vi "Set configuration chain.vi"(8 "error in (no error)":errorcluster, 9 "class names":string[](array[string]), 10 "configuration":variant[](array[variant]), 11 "ExampleClassA in":refnum<class "ExampleClassA.lvclass">) -> (0 "error out":errorcluster, 3 "ExampleClassA out":refnum<class "ExampleClassA.lvclass">)   [LabVIEW 2012, in "ExampleClassA.lvclass"]
uses:
  ExampleClassA.lvclass
  <vilib>/Distrio/Murmex/Murmex/Murmex.lvclass
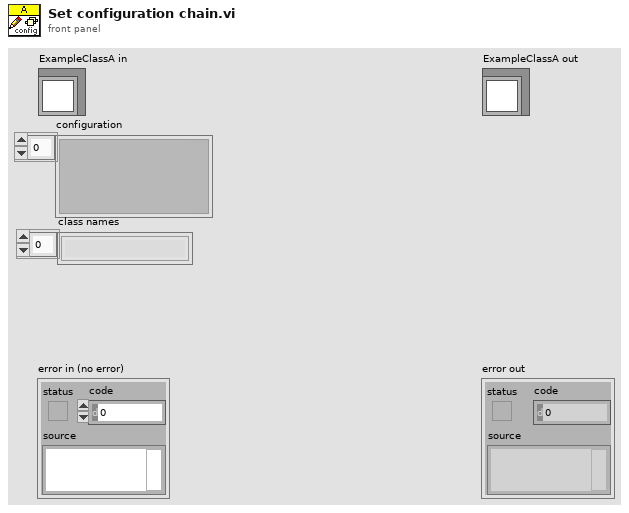
[diagram p1: front panel]
types:
  T1 = typedef "ExampleClassA.lvclass/Settings cluster.ctl" = cluster{"period?":dbl[unit], "number of blocks":i32, "number of channels":i32}
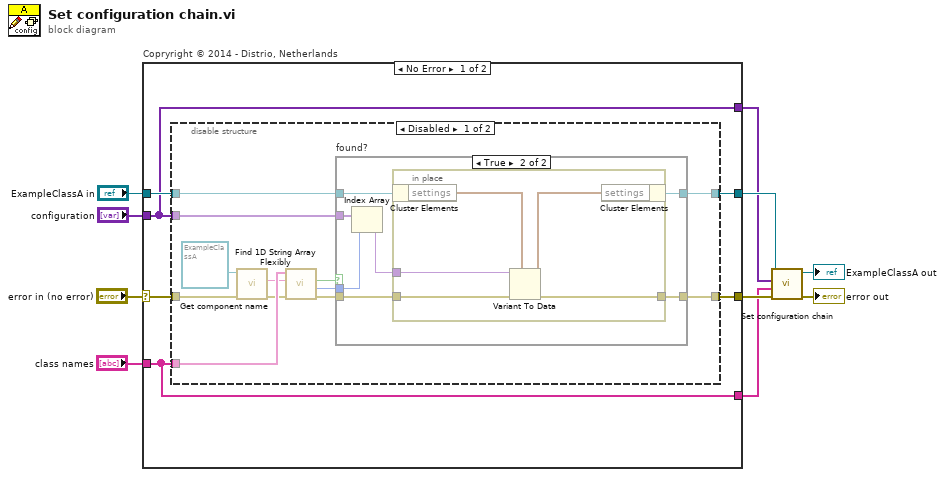
[diagram p0: block diagram]
diagram:
  n1 = case "Copryright © 2014 - Distrio, Netherlands" shown="No Error" "error in (no error)" {
    selector: "error in (no error)" -> [w16 w48]
    tunnel: [w13 w48] -> w8
    tunnel: [w14 w47] -> w3
    tunnel: "ExampleClassA in" -> [w15 w47]
    tunnel: "class names" -> [w11 w45]
    tunnel: "configuration" -> [w12 w46]
    tunnel: [w12 w46] -> w2
    tunnel: [w11 w45] -> w1
    frame No Error {
      n2 = disable-structure shown="Disabled" {
        disable-tunnel: w16 -> [w28 w43]
        disable-tunnel: w15 -> [w18 w44]
        disable-tunnel: [w27 w44] -> w14
        disable-tunnel: [w26 w43] -> w13
        disable-tunnel: w12 -> [w25 _]
        disable-tunnel: w11 -> [w24 _]
        frame Disabled {
          n3 = call <vilib>:"Get component name.vi"("error in (no error)"=w28, "Murmex in"=refnum<class "ExampleClassA.lvclass"> refnum ("ExampleClassA")) -> ("error out"=w22:errorcluster, "component name"=w23:string)  [unwired: 7 in, 1 out]
          n4 = call <vilib>:"Find 1D String Array Flexibly.vi"("error in (no error)"=w22, "element"=w23, "array"=w24) -> ("error out"=w21:errorcluster, "index of element"=w20:i32, "found?"=w19:bool)  [unwired: 6 in]
          n5 = case "found?" shown="True" w19 {
            tunnel: w18 -> [w29 w36]
            tunnel: [w29 w35] -> w27
            tunnel: [w30 w34] -> w26
            tunnel: w25 -> [_ w33]
            tunnel: w21 -> [w30 w32]
            tunnel: w20 -> [_ w31]
            frame False {
            }
            frame True {
              n6 = Index Array(array=w33, index=w31) -> (element=w37:variant)
              n7 = in-place {
                in-place-border: w37 -> [w42]
                in-place-border: w32 -> [w40]
                in-place-border: [w38] -> w34
                n8 = in-place-cluster #1(w36) -> ("settings"=w41:T1)
                n9 = Variant To Data(error in=w40, type=w41, Variant=w42) -> (data=w39:T1, error out=w38:errorcluster)
                n10 = in-place-cluster #1("settings"=w39) -> (w35:refnum<class "ExampleClassA.lvclass">)
              }
            }
          }
        }
        frame Enabled {
        }
      }
    }
    frame Error {
    }
  }
  n11 = call-parent "Set configuration chain.vi"("error in (no error)"=w8, "class names"=w1, "configuration"=w2, "Murmex in"=w3) -> ("error out"=→"error out":errorcluster, "Murmex out"=→"ExampleClassA out":refnum<class "ExampleClassA.lvclass">)  [unwired: 6 in]
